vi "Obtain Data Queue Name.vi"(11 "PackageID":i32) -> (3 "DataQueueName":string)   [LabVIEW 2021, in "XNET-CAN-Signal-Logger.lvlib"]
uses:
  XNET-CAN-Signal-Logger.lvlib
  Global Variables.vi
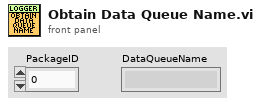
[diagram p1: front panel]
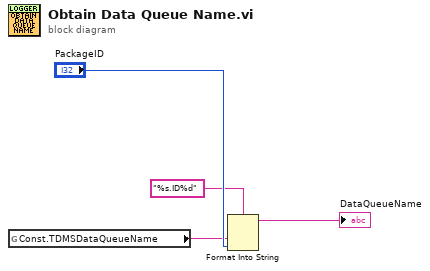
[diagram p0: block diagram]
diagram:
  n1 = global read "Global Variables.vi" "Const.TDMSDataQueueName"() -> (w1:string)
  n2 = Format Into String(format string="%s.ID%d", w1, "PackageID") -> (resulting string=→"DataQueueName":string)  [unwired: 2 in, 1 out]
